vi "VCELoader.vi"   [LabVIEW 2014]
panel:
  # "Launching the Veristand FPGA Configuration Editor..."
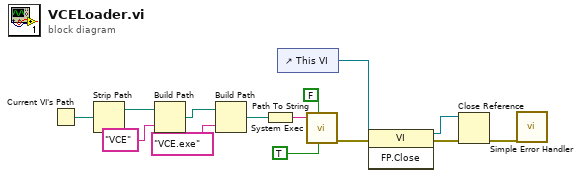
[diagram p0: block diagram]
diagram:
  n1 = Current VI's Path() -> (path=w14:path)
  n2 = Strip Path(path=w14) -> (stripped path=w13:path)  [unwired: 1 out]
  n3 = Build Path(base path=w13, name or relative path="VCE") -> (appended path=w11:path)
  n4 = Build Path(base path=w11, name or relative path="VCE.exe") -> (appended path=w7:path)
  n5 = Path To String(path=w7) -> (string=w8:string)
  n6 = control-ref of="This VI"() -> (w1:refnum<vi>)
  n7 = call <vilib>:"System Exec.vi"("run minimized? (F)"=TRUE, "wait until completion? (T)"=FALSE, "command line"=w8) -> ("error out"=w4:errorcluster)  [unwired: 5 in, 3 out]
  n8 = invoke class="VI" method="FP.Close"(reference=w1, error in=w4) -> (reference out=w2:refnum<vi>, error out=w3:errorcluster)  [unwired: 1 in, 1 out]
  n9 = Close Reference(reference=w2, error in (no error)=w3) -> (error out=w5:errorcluster)
  n10 = call <vilib>:"Simple Error Handler.vi"("error in (no error)"=w5) -> ()  [unwired: 4 in, 5 out]
